vi "Run.vi"(8 "error in (no error)":errorcluster, 9 "s on last turn":dbl, 10 "Maze (0: Empty, -1: Enemy. >0: Teammate":i32[][](array[numeric]), 11 "Expand in":refnum<class "Lone Wolf.lvclass">) -> (0 "error out":errorcluster, 1 "Direction":T1, 2 "Action":T2, 3 "Expand out":refnum<class "Lone Wolf.lvclass">, 4 "Replicated":refnum<class "Square.lvclass">)   [LabVIEW 2015, in "Lone Wolf.lvclass"]
uses:
  Lone Wolf.lvclass
  Type Defs/Action Enum.ctl
  Type Defs/Direction Enum.ctl
  Square/Square.lvclass
  Lone Wolf.lvclass/Lone Wolf.ctl
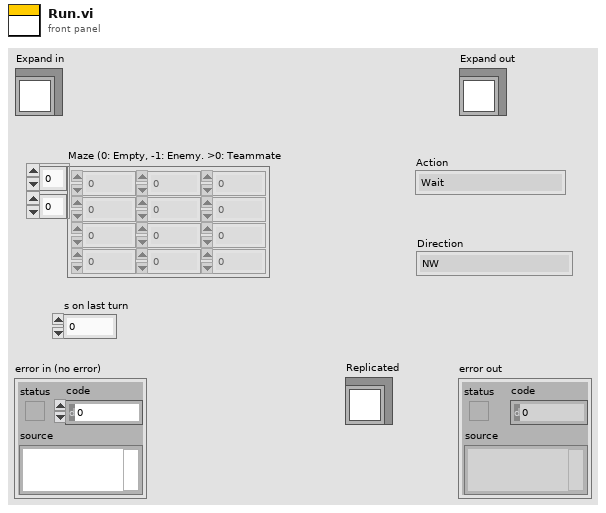
[diagram p1: front panel]
types:
  T1 = typedef "Square.lvclass/Direction Enum.ctl" = enum16{"NW", "N", "NE", "E", "SE", "S", "SW", "W"}
  T2 = typedef "Square.lvclass/Action Enum.ctl" = enum16{"Wait", "Move", "Attack", "Replicate"}
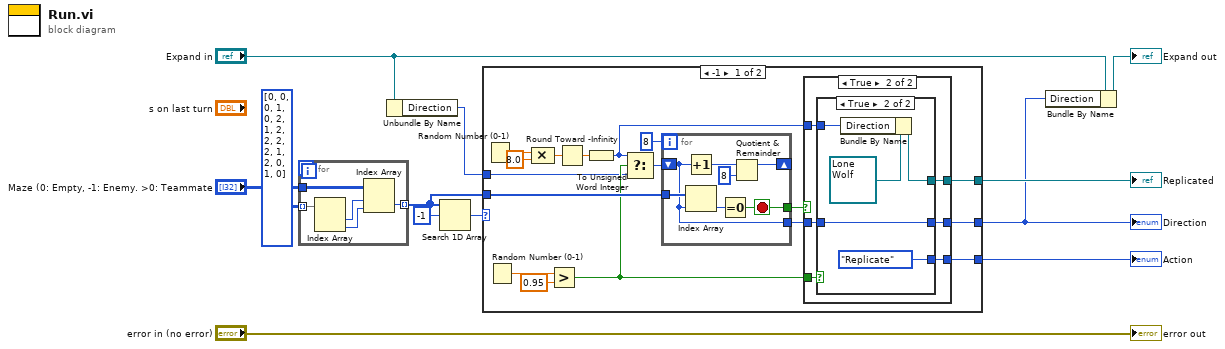
[diagram p0: block diagram]
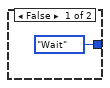
[diagram p2: hidden frame]
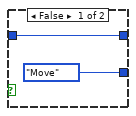
[diagram p3: hidden frame]
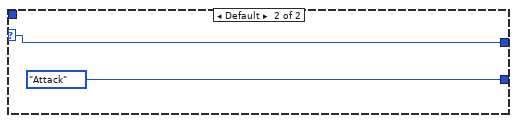
[diagram p4: hidden frame]
diagram:
  n1 = for {
    tunnel: "Maze (0: Empty, -1: Enemy. >0: Teammate" -> [w17]
    tunnel: i32[][] [[0, 0], [0, 1], [0, 2], [1, 2], [2, 2], [2, 1], [2, 0], [1, 0]] -> [w16] mode=indexing
    tunnel: [w13] -> w7 mode=indexing
    n2 = Index Array(array=w16) -> (element #1=w15:i32, element #2=w14:i32)  [unwired: 2 in]
    n3 = Index Array(array=w17, index (row)=w15, index (col)=w14) -> (element=w13:i32)
  }
  n4 = Unbundle By Name("Expand in") -> ("Direction"=w1:T1)
  n5 = Search 1D Array(1D array=w7, element=-1) -> (index of element=w8:i32)  [unwired: 1 in]
  n6 = case shown="-1" w8 {
    selector: w8 -> [_ w56]
    tunnel: [w33 w56] -> w4
    tunnel: [w34 Action_Enum."Attack" ("Action")] -> w5
    tunnel: w7 -> [w28 _]
    tunnel: [w32 _] -> w6
    tunnel: w1 -> [w19 _]
    frame -1 {
      n7 = Random Number (0-1)() -> (number: 0 to 1=w27:dbl)
      n8 = Random Number (0-1)() -> (number: 0 to 1=w30:dbl)
      n9 = Compound Arithmetic op=MULTIPLY(w27, 8.0 ("value")) -> (w25:dbl)
      n10 = Greater?(x=w30, y=0.95) -> (0:w21:bool)
      n11 = Round Toward -Infinity(1:w25) -> (0:w24:dbl)
      n12 = To Unsigned Word Integer(number=w24) -> (unsigned 16bit integer=w18:u16)
      n13 = Select(t=w18, s=w21, f=w19) -> (s? t:f=w20:u16)
      n14 = for {
        N: 8 -> [_]
        tunnel: w28 -> [w55]
        shift-right: [w51] -> _
        shift-left: w20 -> [w50]
        tunnel: [w50] -> w23
        tunnel: [w49] -> w22
        stop <- w49 stop-if-true
        n15 = Increment(x=w50) -> (x+1=w53:i32)
        n16 = Index Array(array=w55, index=w50) -> (element=w54:i32)
        n17 = Equal To 0?(x=w54) -> (x = 0?=w49:bool)
        n18 = Quotient & Remainder(x=w53, y=8) -> (x-y*floor(x/y)=w51:i32)  [unwired: 1 out]
      }
      n19 = case shown="True" w22 {
        tunnel: [Action_Enum."Wait" ("y") w41] -> w34
        tunnel: [_ w40] -> w33
        tunnel: [_ w39] -> w32
        tunnel: w21 -> [_ w38]
        tunnel: w23 -> [_ w37]
        tunnel: w18 -> [_ w36]
        frame False {
        }
        frame True {
          n20 = case shown="True" w38 {
            tunnel: [Action_Enum."Move" ("y") Action_Enum."Replicate" ("y")] -> w41
            tunnel: [w42 w47] -> w40
            tunnel: [_ w44] -> w39
            tunnel: w37 -> [w42 w47]
            tunnel: w36 -> [_ w45]
            frame False {
            }
            frame True {
              n21 = Bundle By Name(cluster=refnum<class "Lone Wolf.lvclass"> refnum ("Lone Wolf.lvclass"), "Direction"=w45) -> (w44:refnum<class "Lone Wolf.lvclass">)
            }
          }
        }
      }
    }
    frame Default {
    }
  }
  "Action" <- w5
  "Direction" <- w4
  "Replicated" <- w6
  n22 = Bundle By Name(cluster="Expand in", "Direction"=w4) -> (→"Expand out":refnum<class "Lone Wolf.lvclass">)
  "error out" <- "error in (no error)"
